vi "measSetToClust.vi"(0 "connection reference":refnum<k7>, 2 "meas_setting def":T2 {"zStartDistCm" format="%.2f"; "numTxCycles" format="%.1f"; "profTxVoltageVolt" format="%#_1g"; "ceilTxVoltageVolt" format="%.2f"; "maxTxVoltageVolt" format="%.2f"; "focusRangeCm" format="%.1f"; "txFrequencyHz" format="%.2f"}, 3 "query results":string[][](array[string]), 4 "floating-point type conversion":string[][](table)=[["extended", "5", "12"], ["double", "5", "9"], ["single", "5", "5"]], 5 "error in":T1) -> (6 "connection reference":refnum<k7>, 7 "meas_setting array":T2[](array[typedef]) {"zStartDistCm" format="%.2f"; "numTxCycles" format="%.1f"; "profTxVoltageVolt" format="%#_1g"; "ceilTxVoltageVolt" format="%.2f"; "maxTxVoltageVolt" format="%.2f"; "focusRangeCm" format="%.1f"; "txFrequencyHz" format="%.2f"}, 8 "error out":T1)   [LabVIEW 2016]
doc: "Takes the query results, a 2D array of strings with a table definition cluster and converts it into an array of clusters of meas_setting. Floating-point conversion has been modified, to use exponential notation for real numbers."
uses:
  type def/measSetting.ctl
panel:
  in  "?":u16[](array[numeric])
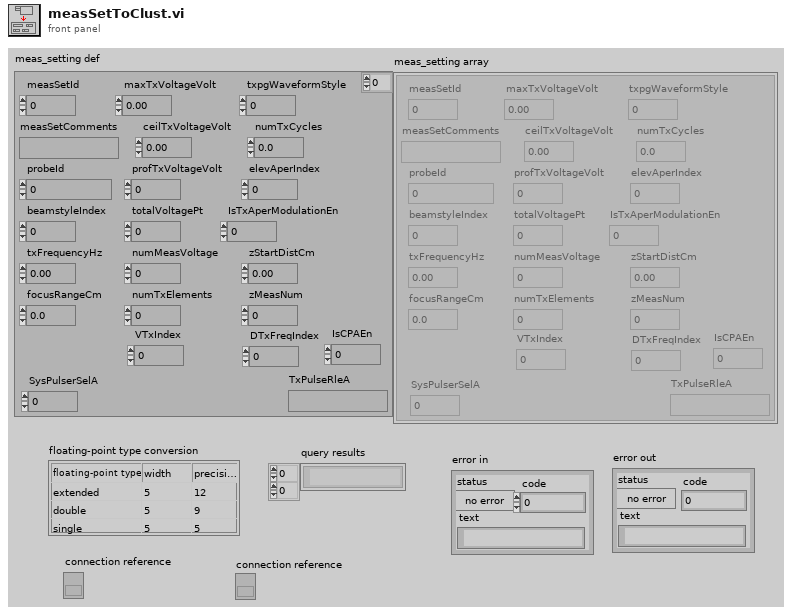
[diagram p1: front panel]
types:
  T1 = cluster{"status":bool, "code":i32, "text":string}
  T2 = typedef "measSetting.ctl" = cluster{"measSetId":i32, "measSetComments":string, "probeId":sgl, "beamstyleIndex":i16, "txFrequencyHz":sgl, "focusRangeCm":sgl, "maxTxVoltageVolt":sgl, "ceilTxVoltageVolt":sgl, "profTxVoltageVolt":dbl, "totalVoltagePt":i8, "numMeasVoltage":i8, "numTxElements":i16, "txpgWaveformStyle":i8, "numTxCycles":sgl, "elevAperIndex":i8, "zStartDistCm":sgl, "zMeasNum":i8, "IsTxAperModulationEn":i8, "DTxFreqIndex":i16, "VTxIndex":i8, "IsCPAEn":i16, "SysPulserSelA":i16, "TxPulseRleA":string}
  T3 = cluster{"name":string, "type  ":u16, "value":string}[]
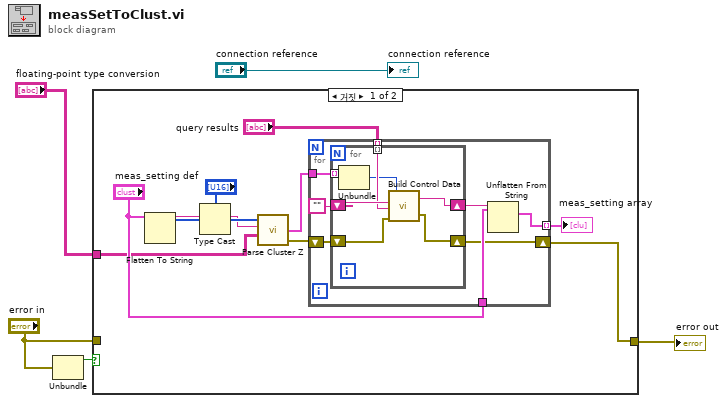
[diagram p0: block diagram]
diagram:
  n1 = Unbundle("error in") -> ("status"=w4:bool)  [unwired: 2 out]
  n2 = case shown="거짓" w4 {
    tunnel: [w8 w32] -> w3
    tunnel: "error in" -> [_ w32]
    tunnel: "floating-point type conversion" -> [w6 _]
    frame False {
      n3 = Flatten To String(anything="meas_setting def") -> (data string=w13:string, type string=w15:i16[])  [unwired: 3 in, 1 out]
      n4 = Type Cast(type="?", x=w15) -> (*(type *) &x=w14:u16[])
      n5 = call "Parse Cluster Z.vi"("floating-point type conversion"=w6, "cluster data"=w13, "cluster definition"=w14) -> ("error out"=w9:T1, "cluster controls"=w10:T3)  [unwired: 1 in, 1 out]
      n6 = for {
        tunnel: [w22] -> w11 mode=indexing
        tunnel: "query results" -> [w21] mode=indexing
        tunnel: w10 -> [w20]
        tunnel: "meas_setting def" -> [w19]
        shift-right: [w17] -> w8
        shift-left: w9 -> [w18]
        n7 = for {
          shift-right: [w30] -> w23
          shift-left: "" -> [w31]
          shift-right: [w28] -> w17
          shift-left: w18 -> [w29]
          tunnel: w21 -> [w27] mode=indexing
          tunnel: w20 -> [w26] mode=indexing
          n8 = Unbundle(w26) -> ("type"=w25:u16)  [unwired: 2 out]
          n9 = call <vilib>:"Build Control Data.vi"("error in"=w29, "cluster data (ascii)"=w27, "cluster data"=w31, "control type"=w25) -> ("error out"=w28:errorcluster, "current cluster data"=w30:string)
        }
        n10 = Unflatten From String(type=w19, binary string=w23) -> (value=w22:T2)  [unwired: 3 in, 2 out]
      }
      "meas_setting array" <- w11
    }
    frame True {
    }
  }
  "error out" <- w3
  "connection reference" <- "connection reference"
